vi "Remove Permission.vi"(8 "error in (no error)":errorcluster, 10 "Label":string, 11 "Topic":refnum<class "Topic.lvclass">) -> (0 "error out":errorcluster, 3 "Topic out":refnum<class "Topic.lvclass">)   [LabVIEW 2015, in "NI_AWS_SNS.lvlib" / "Topic.lvclass"]
uses:
  Topic.lvclass
  Core/HTTP Request/Request Options.ctl
  Core/HTTP Request/Name Value Pair.ctl
  Core/HTTP Request/Region handling.ctl
  Core/HTTP Request/URL formatting.ctl
  Core/ARN/ARN.lvclass/ARN.ctl
  Core/ARN/Read ARN.vi
  Core/HTTP Request/HTTP Request.lvclass
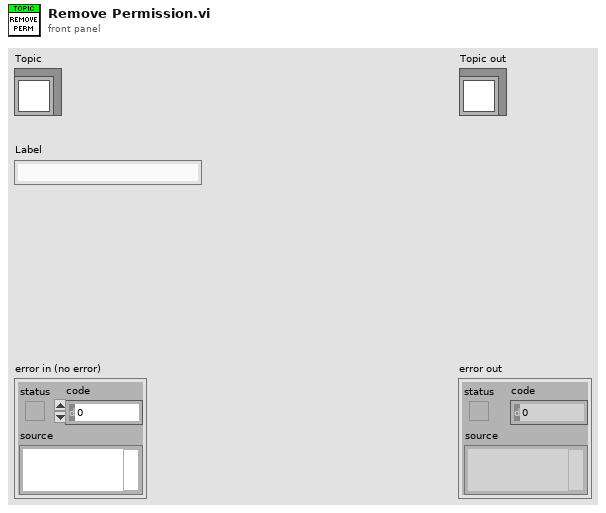
[diagram p1: front panel]
types:
  T1 = typedef "NI_AWS_Core.lvlib/HTTP Request.lvclass/Name Value Pair.ctl" = cluster{"name":string, "value":string}
  T2 = typedef "NI_AWS_Core.lvlib/HTTP Request.lvclass/Request Options.ctl" = cluster{"request headers":T1[], "request parameters":T1[], "request body":string, "region handling":T3, "URL formatting":T4}
  T3 = typedef "NI_AWS_Core.lvlib/HTTP Request.lvclass/Region handling.ctl" = enum16{"use region everywhere", "use region (authentication only)", "use region (URL only)", "ignore region everwhere"}
  T4 = typedef "NI_AWS_Core.lvlib/HTTP Request.lvclass/URL formatting.ctl" = enum16{"region-", "region."}
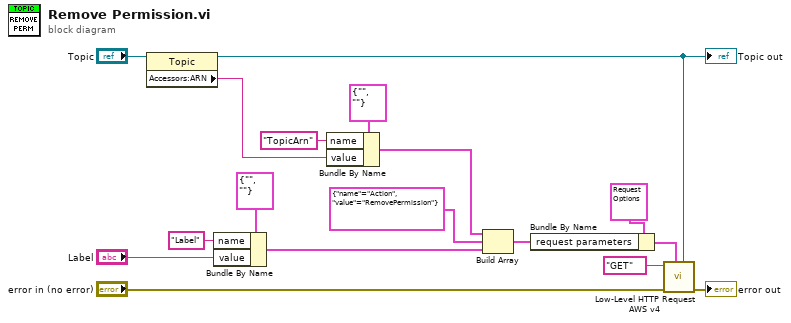
[diagram p0: block diagram]
diagram:
  n1 = property class="Topic"(reference="Topic") -> (reference out=w11:refnum<class "Topic.lvclass">, "Accessors:ARN"=w6:string)  [unwired: 1 in, 1 out]
  "Topic out" <- w11
  n2 = Bundle By Name(cluster=T1 {"name"="", "value"=""} ("element"), "name"="Label", "value"="Label") -> (w1:T1)
  n3 = Bundle By Name(cluster=T1 {"name"="", "value"=""} ("element"), "name"="TopicArn", "value"=w6) -> (w5:T1)
  n4 = Build Array(w5, T1 {"name"="Action", "value"="RemovePermission"} ("Cluster"), w1) -> (w9:T1[])
  n5 = Bundle By Name(cluster=T2 {"request headers"=[], "request parameters"=[{"name"="Action", "value"="ListQueues"}], "request body"="", "region handling"=enum."use region everywhere", "URL formatting"=enum."region."} ("Request Options"), "request parameters"=w9) -> (w12:T2)
  n6 = call "Low-Level HTTP Request AWS v4.vi"("AWS Core"=w11, "Request Options"=w12, "error in (no error)"="error in (no error)", "HTTP-Verb"="GET") -> ("error out"=→"error out":errorcluster)  [unwired: 5 in, 2 out]
